vi "SUB-BLE Rx data (Mon)-CDC IMU.vi"(8 "data in":u8[](array[numeric]) format="%2x") -> (0 "IMU data":T1 caption="IMU Monitoring data" {"Accelerometer Z" format="%#.9f"; "Accelerometer Y" format="%#.9f"; "Accelerometer X" format="%#.9f"; "Gyroscope Z" format="%#.9f"; "Gyroscope Y" format="%#.9f"; "Gyroscope X" format="%#.9f"}, 1 "CDC data":T2 caption="CDC Monitoring data" {"Right Wing-C, C6/C0" format="%#.9f"; "Right Wing-B, C5/C0" format="%#.9f"; "Right Wing-A, C4/C0" format="%#.9f"; "Left Wing-C, C3/C0" format="%#.9f"; "Left Wing-B, C2/C0" format="%#.9f"; "Left Wing-A, C1/C0" format="%#.9f"}, 2 "Bat":u16, 3 "*Board ID":string="None...." caption="S/N")   [LabVIEW 2015]
doc: "Use this template to create an application that executes repeatedly until you click the Stop button. This template polls the state of the Stop button and does not use events. Use the Top-Level Application template (not available in the Base package) to create a single-loop application with event handling."
uses:
  Control-CDC data.ctl
  Control-IMU data.ctl
panel:
  out "BLE Packet (buf)":u8[](array[numeric])
  out "BLE Packet (data)":u8[](array[numeric])
  # "BLE 수신 데이터를 분류: Monitoring/Setting data"
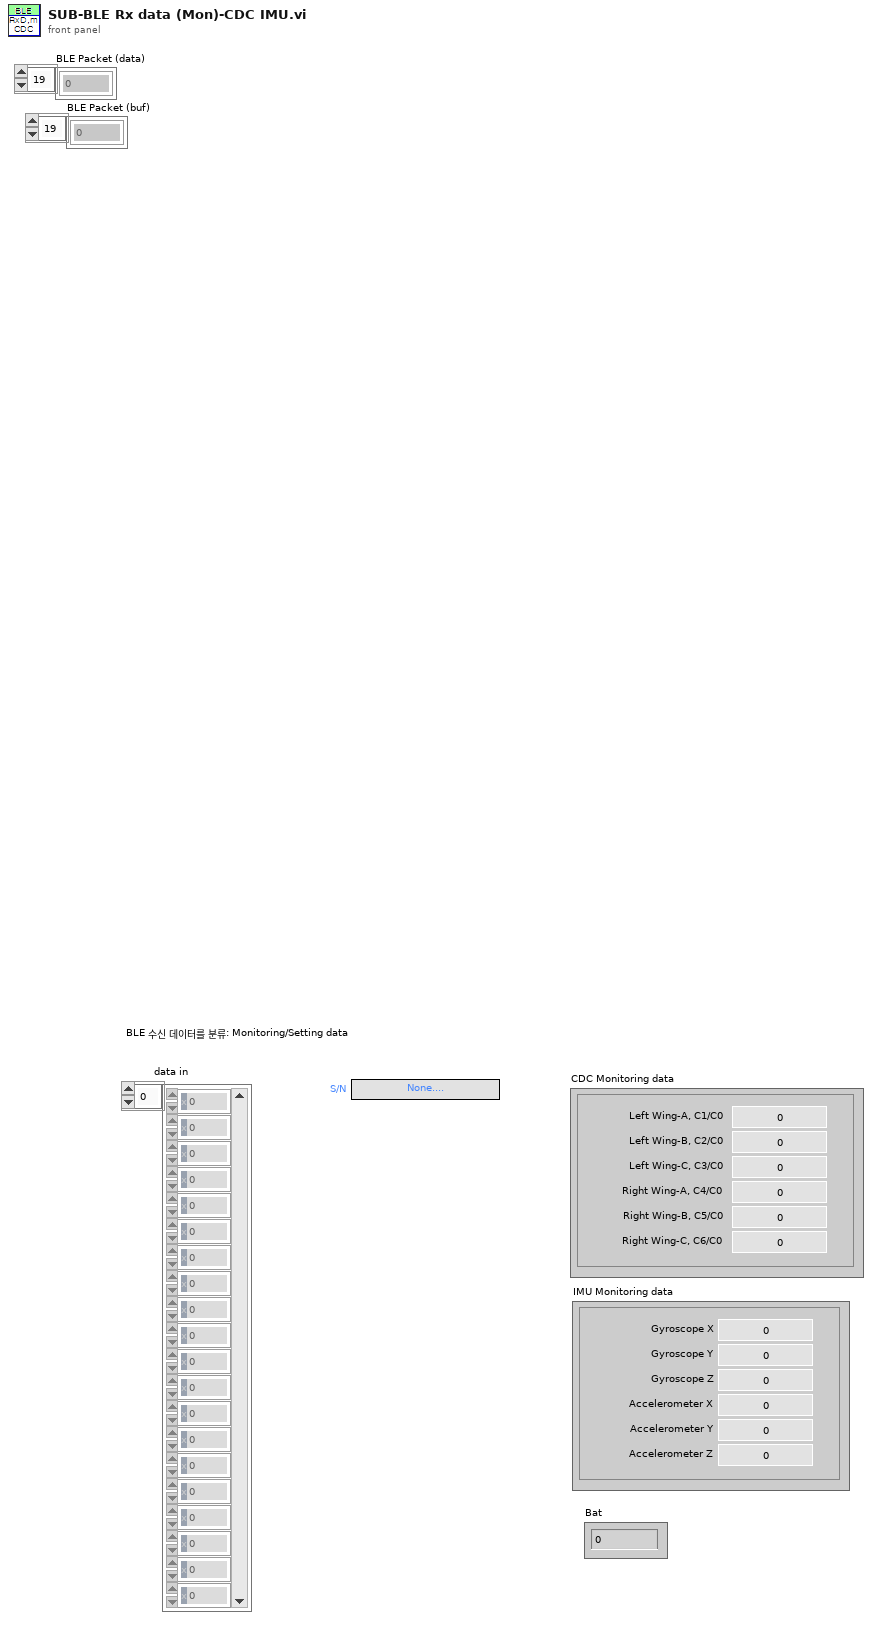
[diagram p1: front panel]
types:
  T1 = typedef "Control-IMU data.ctl" = cluster{"Gyroscope X":dbl, "Gyroscope Y":dbl, "Gyroscope Z":dbl, "Accelerometer X":dbl, "Accelerometer Y":dbl, "Accelerometer Z":dbl}
  T2 = typedef "Control-CDC data.ctl" = cluster{"Left Wing-A, C1/C0":dbl, "Left Wing-B, C2/C0":dbl, "Left Wing-C, C3/C0":dbl, "Right Wing-A, C4/C0":dbl, "Right Wing-B, C5/C0":dbl, "Right Wing-C, C6/C0":dbl}
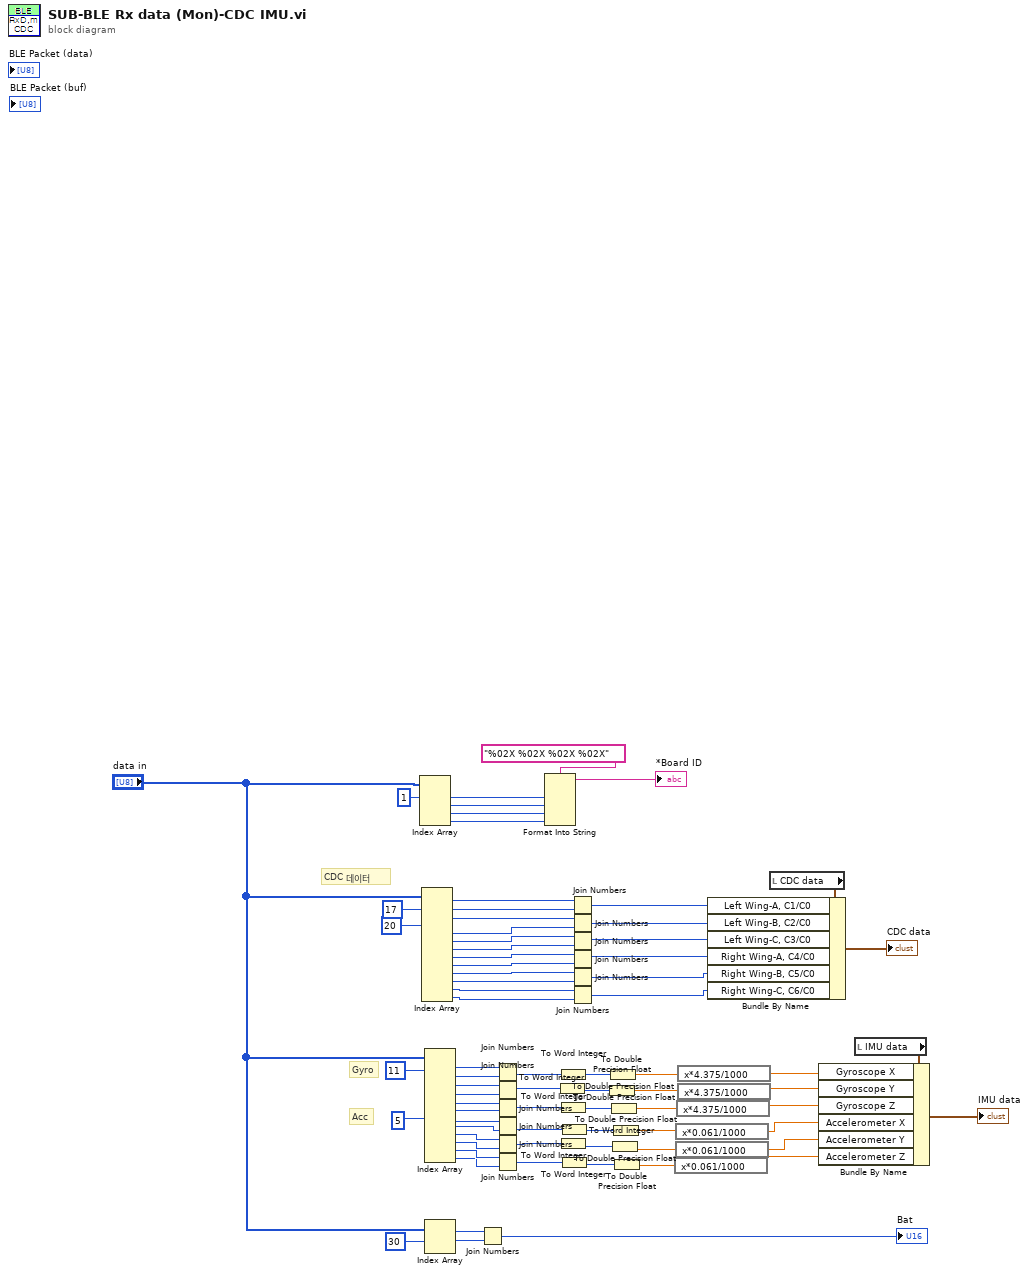
[diagram p0: block diagram]
diagram:
  # "Acc"
  # "Gyro"
  # "CDC 데이터"
  n1 = Index Array(array="data in", index #1=1 ("인덱스")) -> (element #1=w72:u8, element #2=w71:u8, element #3=w70:u8, element #4=w69:u8)  [unwired: 3 in]
  n2 = Index Array(array="data in", index #1=17 ("인덱스"), index #3=20 ("인덱스")) -> (element #1=w65:u8, element #2=w64:u8, element #3=w63:u8, element #4=w62:u8, element #5=w61:u8, element #6=w60:u8, element #7=w59:u8, element #8=w58:u8, element #9=w57:u8, element #10=w56:u8, element #11=w55:u8, element #12=w54:u8)  [unwired: 10 in]
  n3 = Index Array(array="data in", index #1=11 ("인덱스"), index #7=5 ("인덱스")) -> (element #1=w43:u8, element #2=w42:u8, element #3=w41:u8, element #4=w40:u8, element #5=w39:u8, element #6=w38:u8, element #7=w37:u8, element #8=w36:u8, element #9=w35:u8, element #10=w34:u8, element #11=w33:u8, element #12=w32:u8)  [unwired: 10 in]
  n4 = Index Array(array="data in", index #1=30 ("인덱스")) -> (element #1=w16:u8, element #2=w17:u8)  [unwired: 1 in]
  n5 = Join Numbers(hi=w16, lo=w17) -> ((hi.lo)=→"Bat":u16)
  n6 = Join Numbers(hi=w43, lo=w42) -> ((hi.lo)=w6:u16)
  n7 = Join Numbers(hi=w41, lo=w40) -> ((hi.lo)=w5:u16)
  n8 = Join Numbers(hi=w39, lo=w38) -> ((hi.lo)=w4:u16)
  n9 = Join Numbers(hi=w37, lo=w36) -> ((hi.lo)=w3:u16)
  n10 = Join Numbers(hi=w35, lo=w34) -> ((hi.lo)=w2:u16)
  n11 = Join Numbers(hi=w33, lo=w32) -> ((hi.lo)=w1:u16)
  n12 = Format Into String(format string="%02X %02X %02X %02X" ("구분 문자(탭)"), w72, w71, w70, w69) -> (resulting string=→"*Board ID":string)  [unwired: 2 in, 1 out]
  n13 = To Word Integer(number=w5) -> (16bit integer=w8:i16)
  n14 = To Word Integer(number=w6) -> (16bit integer=w7:i16)
  n15 = To Word Integer(number=w4) -> (16bit integer=w9:i16)
  n16 = To Word Integer(number=w2) -> (16bit integer=w11:i16)
  n17 = To Word Integer(number=w3) -> (16bit integer=w12:i16)
  n18 = To Word Integer(number=w1) -> (16bit integer=w10:i16)
  n19 = Join Numbers(hi=w65, lo=w64) -> ((hi.lo)=w51:u16)
  n20 = Join Numbers(hi=w63, lo=w62) -> ((hi.lo)=w50:u16)
  n21 = Join Numbers(hi=w61, lo=w60) -> ((hi.lo)=w49:u16)
  n22 = Join Numbers(hi=w59, lo=w58) -> ((hi.lo)=w48:u16)
  n23 = Join Numbers(hi=w57, lo=w56) -> ((hi.lo)=w47:u16)
  n24 = Join Numbers(hi=w55, lo=w54) -> ((hi.lo)=w46:u16)
  n25 = To Double Precision Float(number=w8) -> (double precision float=w25:dbl)
  n26 = To Double Precision Float(number=w7) -> (double precision float=w30:dbl)
  n27 = To Double Precision Float(number=w9) -> (double precision float=w26:dbl)
  n28 = To Double Precision Float(number=w11) -> (double precision float=w28:dbl)
  n29 = To Double Precision Float(number=w12) -> (double precision float=w29:dbl)
  n30 = To Double Precision Float(number=w10) -> (double precision float=w27:dbl)
  n31 = expression code="x*0.061/1000"(w27) -> (w18:dbl)
  n32 = expression code="x*0.061/1000"(w29) -> (w20:dbl)
  n33 = expression code="x*0.061/1000"(w28) -> (w19:dbl)
  n34 = expression code="x*4.375/1000"(w26) -> (w21:dbl)
  n35 = expression code="x*4.375/1000"(w30) -> (w23:dbl)
  n36 = expression code="x*4.375/1000"(w25) -> (w22:dbl)
  n37 = local read "CDC data"() -> (w67:T2)
  n38 = Bundle By Name(cluster=w67, "Left Wing-A, C1/C0"=w51, "Left Wing-B, C2/C0"=w50, "Left Wing-C, C3/C0"=w49, "Right Wing-A, C4/C0"=w48, "Right Wing-B, C5/C0"=w47, "Right Wing-C, C6/C0"=w46) -> (→"CDC data":T2)
  n39 = local read "IMU data"() -> (w45:T1)
  n40 = Bundle By Name(cluster=w45, "Gyroscope X"=w23, "Gyroscope Y"=w22, "Gyroscope Z"=w21, "Accelerometer X"=w20, "Accelerometer Y"=w19, "Accelerometer Z"=w18) -> (→"IMU data":T1)
